vi "String2Hex.vi"(1 "value":string) -> (0 "String":string)   [LabVIEW 2010]
panel:
  out "substring":string
  out "String 2":string
  out "data string":string
  out "length 3":i32
  out "value 2":string
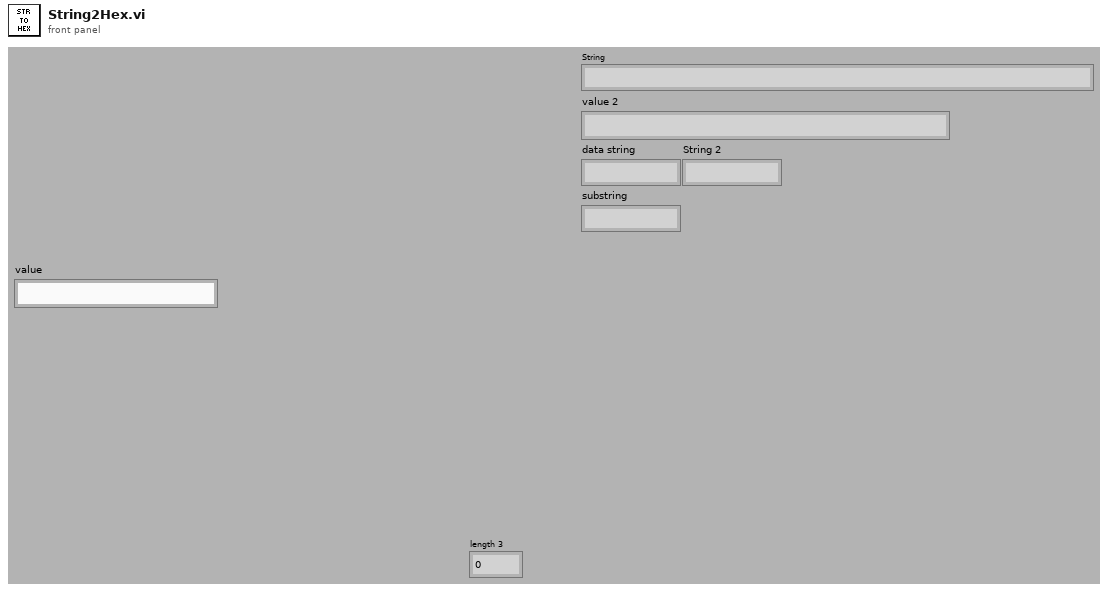
[diagram p1: front panel]
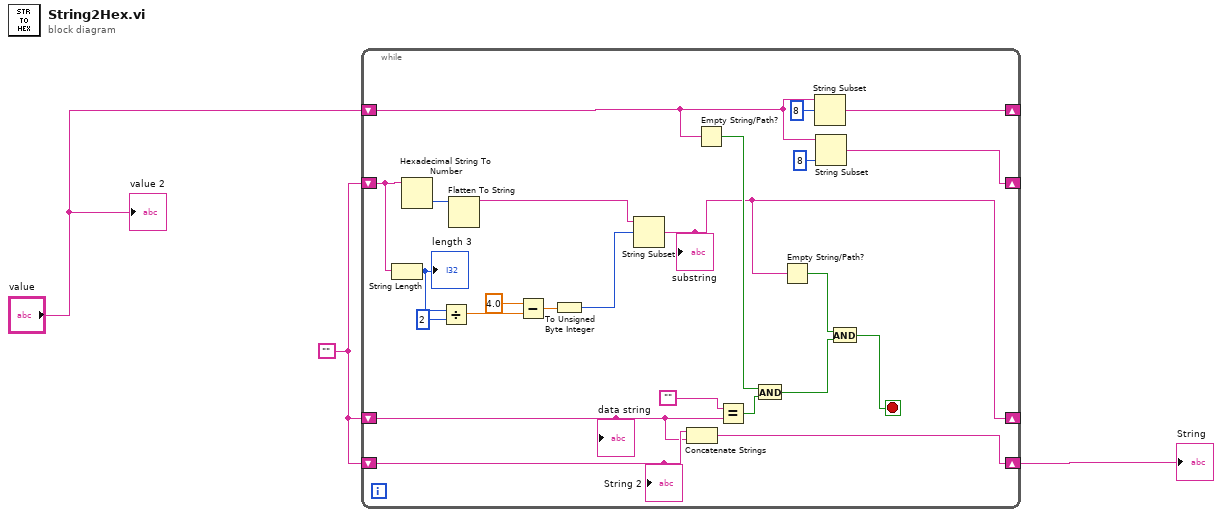
[diagram p0: block diagram]
diagram:
  w1 = ""
  n1 = while {
    shift-right: [w25] -> _
    shift-left: "value" -> [w21]
    shift-right: [w24] -> _
    shift-left: w1 -> [w12]
    shift-right: [w7] -> _
    shift-left: w1 -> [w8]
    shift-right: [w22] -> w2
    shift-left: w1 -> [w18]
    stop <- w4 stop-if-true
    n2 = String Length(string=w12) -> (length=w13:i32)
    "length 3" <- w13
    n3 = Hexadecimal String To Number(string=w12) -> (number=w23:u32)  [unwired: 2 in, 1 out]
    n4 = Divide(x=w13, y=2) -> (x/y=w16:dbl)
    n5 = Flatten To String(anything=w23) -> (data string=w10:string)  [unwired: 3 in, 2 out]
    n6 = Subtract(x=4.0, y=w16) -> (x-y=w17:dbl)
    n7 = To Unsigned Byte Integer(number=w17) -> (unsigned 8bit integer=w11:u8)
    n8 = String Subset(string=w10, offset (0)=w11) -> (substring=w7:string)  [unwired: 1 in]
    "substring" <- w7
    n9 = Concatenate Strings(w18, w8) -> (w22:string)
    n10 = Empty String/Path?(string/path=w21) -> (empty?=w19:bool)
    n11 = Equal?(x="", y=w8) -> (x = y?=w20:bool)
    n12 = And(x=w19, y=w20) -> (x .and. y?=w6:bool)
    n13 = Empty String/Path?(string/path=w7) -> (empty?=w5:bool)
    n14 = String Subset(string=w21, offset (0)=8 ("length (rest)")) -> (substring=w25:string)  [unwired: 1 in]
    n15 = String Subset(string=w21, length (rest)=8 ("length (rest)")) -> (substring=w24:string)  [unwired: 1 in]
    n16 = And(x=w5, y=w6) -> (x .and. y?=w4:bool)
    "data string" <- w8
    "String 2" <- w18
  }
  "String" <- w2
  "value 2" <- "value"
